vi "stop seq.vi"(8 "error in (no error)":errorcluster) -> (0 "error out":errorcluster)   [LabVIEW 2019]
uses:
  ctl/servo act.ctl
  FPGA_subVIs/low level/DIO/DIO enum.ctl
  FPGA_subVIs/low level/DIO/DIO.lvclass
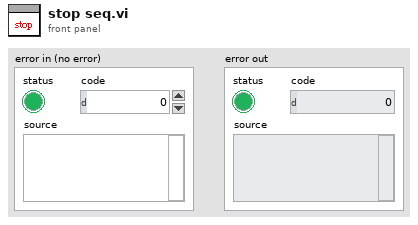
[diagram p1: front panel]
types:
  T1 = typedef "servo act.ctl" = enum16{"catch", "relax", "left idle", "center", "red relax", "left reg", "right reg"}
  T2 = typedef "my FPGA lib.lvlib/DIO.lvclass/DIO enum.ctl" = enum16{"US.1", "US.2", "US.3", "US.4", "H.1", "H.2", "H.3", "H.4", "H.5"}
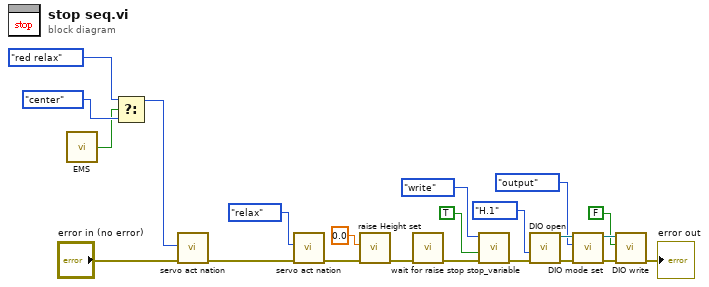
[diagram p0: block diagram]
diagram:
  n1 = call "EMS.vi"() -> ("A/DIO4 (Pin 19)"=w1:bool)
  n2 = Select(t=servo_act."red relax" ("servo act"), s=w1, f=servo_act."center" ("servo act")) -> (s? t:f=w4:T1)
  n3 = call "servo act nation.vi"("error in"="error in (no error)", "servo act"=w4) -> ("error out"=w16:errorcluster)  [unwired: 9 in]
  n4 = call "servo act nation.vi"("error in"=w16, "servo act"=servo_act."relax") -> ("error out"=w14:errorcluster)  [unwired: 9 in]
  n5 = call "raise Height set.vi"("error in (no error)"=w14, "Height_cm"=0.0) -> ("error out"=w20:errorcluster)  [unwired: 9 in]
  n6 = call "wait for raise stop.vi"("Error In"=w20) -> ("Error Out"=w18:errorcluster)  [unwired: 10 in]
  n7 = call "stop_variable.vi"("Error In"=w18, "Write"=TRUE, "Enum"=enum16{"read", "write"}."write") -> ("Error Out"=w5:errorcluster)  [unwired: 7 in, 1 out]
  n8 = call "DIO open.vi"("error in"=w5, "DIO reference"=DIO_enum."H.1") -> ("error out"=w13:errorcluster, "my FPGA lib.lvlib:DIO.lvclass"=w12:refnum<class "DIO.lvclass">)  [unwired: 8 in]
  n9 = call "DIO mode set.vi"("error in (no error)"=w13, "mode"=enum16{"input", "output"}."output", "DIO in"=w12) -> ("error out"=w9:errorcluster, "DIO out"=w8:refnum<class "DIO.lvclass">)  [unwired: 7 in]
  n10 = call-dynamic "DIO write.vi"("error in (no error)"=w9, "output"=FALSE, "DIO in"=w8) -> ("error out"=→"error out":errorcluster)  [unwired: 7 in, 1 out]
